vi "Is Asynchronous Call.vi"() -> (0 "Async Call?":bool)   [LabVIEW 2017, in "CSM Shared.lvlib"]
uses:
  CSM Shared.lvlib
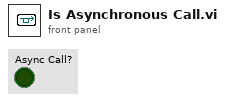
[diagram p1: front panel]
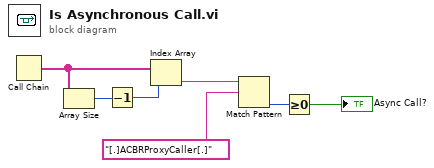
[diagram p0: block diagram]
diagram:
  n1 = Call Chain() -> (call chain=w6:string[])
  n2 = Array Size(array=w6) -> (size(s)=w7:i32)
  n3 = Decrement(x=w7) -> (x-1=w5:i32)
  n4 = Index Array(array=w6, index=w5) -> (element=w4:string)
  n5 = Match Pattern(string=w4, regular expression="[.]ACBRProxyCaller[.]") -> (offset past match=w2:i32)  [unwired: 1 in, 3 out]
  n6 = Greater Or Equal To 0?(x=w2) -> (x >= 0?=→"Async Call?":bool)
